vi "VI Tree.vi"   [LabVIEW 2020, in "NH Research Regenerative Test Series.lvlib"]
doc: "This instrument driver supports the NH Research 9400 Series AC/DC Power Module\".\n<B>Model Number</B> : 9400-4, 9400-8, 9400-12, 9400-24, 9400-36, 9400-48, 9400-64, 9400-96.\n\nThe VI Tree displays all the user-callable VIs of the instrument driver in an organized table."
uses:
  Drivers-Essentials/NH Research Regenerative Test Series.lvlib
  <instrlib>/NH Research Regenerative Test Series/Public/Data/Low Level/Fetch Array (Current).vi
  <instrlib>/NH Research Regenerative Test Series/Public/Data/Low Level/Fetch Waveform (Voltage).vi
  <instrlib>/NH Research Regenerative Test Series/Public/Data/Read Waveform (Voltage).vi
  <instrlib>/NH Research Regenerative Test Series/Public/Data/Read Array (Current).vi
  Data/Low Level/Fetch (Ave Current).vi
  Configure/Configure Slew Rate (Voltage).vi
  Action-Status/Query Slew Rate (Voltage).vi
  Action-Status/Reset Measurements (All).vi
  Data/Fetch Background Measurements (Basic).vi
  Drivers-Essentials/Read (Ave Current).vi
  Utility/Query Capabilities (Voltage).vi
panel:
  # "SEE DIAGRAM\nFOR VI TREE."
  # "NH Research, Inc. \n16601 Hale Avenue\nIrvine, CA 92606\n\nPhone:    (949) 474-3900\nEmail:      sales@nhresearch.com"
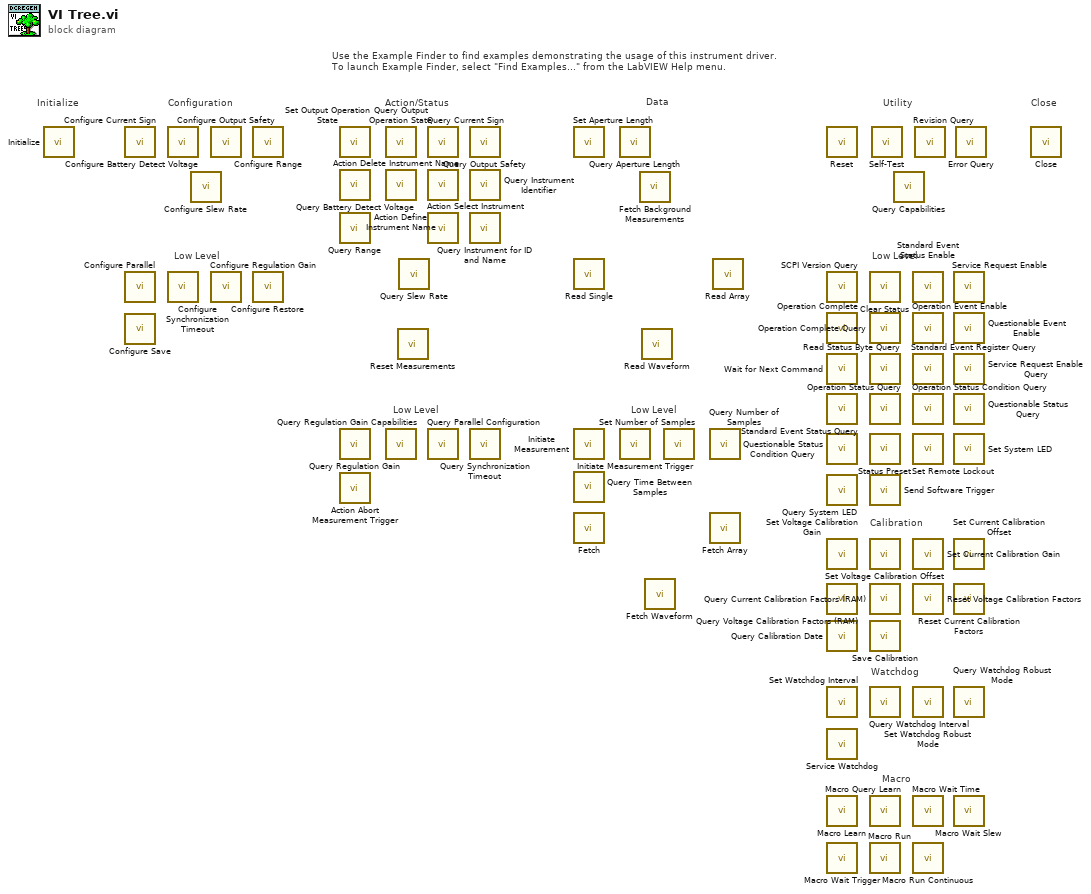
[diagram p0: block diagram]
diagram:
  # "Macro"
  # "Watchdog"
  # "Low Level"
  # "Calibration"
  # "Low Level"
  # "Low Level"
  # "Use the Example Finder to find examples demonstrating the usage of this instrument driver.\nTo launch Example Finder, select \"Find Examples...\" from the LabVIEW Help menu."
  # "Low Level"
  # "Configuration"
  # "Utility"
  # "Data"
  # "Action/Status"
  # "Close"
  # "Initialize"
  n1 = call <instrlib>:"Initialize.vi"() -> ()  [unwired: 14 in, 2 out]
  n2 = call <instrlib>:"Configure Current Sign.vi"() -> ()  [unwired: 14 in, 2 out]
  n3 = call <instrlib>:"Configure Parallel.vi"() -> ()  [unwired: 14 in, 2 out]
  n4 = call <instrlib>:"Configure Save.vi"() -> ()  [unwired: 14 in, 2 out]
  n5 = call "Configure Battery Detect Voltage.vi"() -> ()  [unwired: 14 in, 2 out]
  n6 = call <instrlib>:"Configure Synchronization Timeout.vi"() -> ()  [unwired: 14 in, 2 out]
  n7 = call-poly <instrlib>:"Configure Slew Rate.vi"() -> ()  [unwired: 14 in, 2 out]
  n8 = call <instrlib>:"Configure Output Safety.vi"() -> ()  [unwired: 14 in, 2 out]
  n9 = call <instrlib>:"Configure Regulation Gain.vi"() -> ()  [unwired: 14 in, 2 out]
  n10 = call "Configure Range.vi"() -> ()  [unwired: 14 in, 2 out]
  n11 = call <instrlib>:"Configure Restore.vi"() -> ()  [unwired: 14 in, 2 out]
  n12 = call <instrlib>:"Set Output Operation State.vi"() -> ()  [unwired: 14 in, 2 out]
  n13 = call <instrlib>:"Query Battery Detect Voltage.vi"() -> ()  [unwired: 13 in, 3 out]
  n14 = call "Query Range.vi"() -> ()  [unwired: 13 in, 3 out]
  n15 = call <instrlib>:"Query Regulation Gain.vi"() -> ()  [unwired: 13 in, 3 out]
  n16 = call <instrlib>:"Action Abort Measurement Trigger.vi"() -> ()  [unwired: 14 in, 2 out]
  n17 = call <instrlib>:"Query Output Operation State.vi"() -> ()  [unwired: 8 in, 8 out]
  n18 = call <instrlib>:"Action Define Instrument Name.vi"() -> ()  [unwired: 14 in, 2 out]
  n19 = call <instrlib>:"Query Regulation Gain Capabilities.vi"() -> ()  [unwired: 11 in, 5 out]
  n20 = call-poly <instrlib>:"Reset Measurements.vi"() -> ()  [unwired: 14 in, 2 out]
  n21 = call-poly <instrlib>:"Query Slew Rate.vi"() -> ()  [unwired: 13 in, 3 out]
  n22 = call "Query Current Sign.vi"() -> ()  [unwired: 13 in, 3 out]
  n23 = call <instrlib>:"Action Delete Instrument Name.vi"() -> ()  [unwired: 14 in, 2 out]
  n24 = call <instrlib>:"Action Select Instrument.vi"() -> ()  [unwired: 14 in, 2 out]
  n25 = call "Query Parallel Configuration.vi"() -> ()  [unwired: 13 in, 3 out]
  n26 = call "Query Output Safety.vi"() -> ()  [unwired: 13 in, 3 out]
  n27 = call <instrlib>:"Query Instrument Identifier.vi"() -> ()  [unwired: 13 in, 3 out]
  n28 = call <instrlib>:"Query Instrument for ID and Name.vi"() -> ()  [unwired: 12 in, 4 out]
  n29 = call "Query Synchronization Timeout.vi"() -> ()  [unwired: 13 in, 3 out]
  n30 = call <instrlib>:"Set Aperture Length.vi"() -> ()  [unwired: 14 in, 2 out]
  n31 = call-poly <instrlib>:"Read Single.vi"() -> ()  [unwired: 13 in, 3 out]
  n32 = call <instrlib>:"Initiate Measurement.vi"() -> ()  [unwired: 14 in, 2 out]
  n33 = call <instrlib>:"Query Time Between Samples.vi"() -> ()  [unwired: 13 in, 3 out]
  n34 = call-poly <instrlib>:"Fetch.vi"() -> ()  [unwired: 13 in, 3 out]
  n35 = call <instrlib>:"Query Aperture Length.vi"() -> ()  [unwired: 13 in, 3 out]
  n36 = call "Initiate Measurement Trigger.vi"() -> ()  [unwired: 14 in, 2 out]
  n37 = call-poly "Fetch Background Measurements.vi"() -> ()  [unwired: 13 in, 3 out]
  n38 = call-poly <instrlib>:"Read Waveform.vi"() -> ()  [unwired: 13 in, 3 out]
  n39 = call-poly <instrlib>:"Fetch Waveform.vi"() -> ()  [unwired: 13 in, 3 out]
  n40 = call <instrlib>:"Set Number of Samples.vi"() -> ()  [unwired: 14 in, 2 out]
  n41 = call <instrlib>:"Query Number of Samples.vi"() -> ()  [unwired: 13 in, 3 out]
  n42 = call-poly <instrlib>:"Fetch Array.vi"() -> ()  [unwired: 13 in, 3 out]
  n43 = call-poly <instrlib>:"Read Array.vi"() -> ()  [unwired: 13 in, 3 out]
  n44 = call <instrlib>:"Reset.vi"() -> ()  [unwired: 14 in, 2 out]
  n45 = call <instrlib>:"SCPI Version Query.vi"() -> ()  [unwired: 13 in, 3 out]
  n46 = call <instrlib>:"Operation Complete.vi"() -> ()  [unwired: 14 in, 2 out]
  n47 = call <instrlib>:"Wait for Next Command.vi"() -> ()  [unwired: 14 in, 2 out]
  n48 = call <instrlib>:"Standard Event Status Query.vi"() -> ()  [unwired: 13 in, 3 out]
  n49 = call <instrlib>:"Questionable Status Condition Query.vi"() -> ()  [unwired: 13 in, 3 out]
  n50 = call <instrlib>:"Query System LED.vi"() -> ()  [unwired: 13 in, 3 out]
  n51 = call "Set Voltage Calibration Gain.vi"() -> ()  [unwired: 14 in, 2 out]
  n52 = call <instrlib>:"Query Voltage Calibration Factors (RAM).vi"() -> ()  [unwired: 13 in, 3 out]
  n53 = call <instrlib>:"Query Calibration Date.vi"() -> ()  [unwired: 13 in, 3 out]
  n54 = call <instrlib>:"Set Watchdog Interval.vi"() -> ()  [unwired: 14 in, 2 out]
  n55 = call <instrlib>:"Service Watchdog.vi"() -> ()  [unwired: 14 in, 2 out]
  n56 = call "Macro Learn.vi"() -> ()  [unwired: 14 in, 2 out]
  n57 = call "Macro Wait Trigger.vi"() -> ()  [unwired: 14 in, 2 out]
  n58 = call <instrlib>:"Clear Status.vi"() -> ()  [unwired: 14 in, 2 out]
  n59 = call <instrlib>:"Operation Complete Query.vi"() -> ()  [unwired: 13 in, 3 out]
  n60 = call <instrlib>:"Read Status Byte Query.vi"() -> ()  [unwired: 13 in, 3 out]
  n61 = call <instrlib>:"Operation Status Query.vi"() -> ()  [unwired: 13 in, 3 out]
  n62 = call <instrlib>:"Status Preset.vi"() -> ()  [unwired: 14 in, 2 out]
  n63 = call "Send Software Trigger.vi"() -> ()  [unwired: 14 in, 2 out]
  n64 = call "Set Voltage Calibration Offset.vi"() -> ()  [unwired: 14 in, 2 out]
  n65 = call <instrlib>:"Query Current Calibration Factors (RAM).vi"() -> ()  [unwired: 13 in, 3 out]
  n66 = call <instrlib>:"Save Calibration.vi"() -> ()  [unwired: 14 in, 2 out]
  n67 = call <instrlib>:"Query Watchdog Interval.vi"() -> ()  [unwired: 13 in, 3 out]
  n68 = call "Macro Query Learn.vi"() -> ()  [unwired: 13 in, 3 out]
  n69 = call "Macro Run.vi"() -> ()  [unwired: 14 in, 2 out]
  n70 = call <instrlib>:"Self-Test.vi"() -> ()  [unwired: 13 in, 3 out]
  n71 = call-poly <instrlib>:"Query Capabilities.vi"() -> ()  [unwired: 13 in, 3 out]
  n72 = call <instrlib>:"Standard Event Status Enable.vi"() -> ()  [unwired: 14 in, 2 out]
  n73 = call <instrlib>:"Operation Event Enable.vi"() -> ()  [unwired: 14 in, 2 out]
  n74 = call <instrlib>:"Standard Event Register Query.vi"() -> ()  [unwired: 13 in, 3 out]
  n75 = call <instrlib>:"Operation Status Condition Query.vi"() -> ()  [unwired: 13 in, 3 out]
  n76 = call <instrlib>:"Set Remote Lockout.vi"() -> ()  [unwired: 14 in, 2 out]
  n77 = call <instrlib>:"Set Current Calibration Gain.vi"() -> ()  [unwired: 14 in, 2 out]
  n78 = call <instrlib>:"Reset Voltage Calibration Factors.vi"() -> ()  [unwired: 14 in, 2 out]
  n79 = call <instrlib>:"Set Watchdog Robust Mode.vi"() -> ()  [unwired: 14 in, 2 out]
  n80 = call "Macro Wait Time.vi"() -> ()  [unwired: 14 in, 2 out]
  n81 = call "Macro Run Continuous.vi"() -> ()  [unwired: 14 in, 2 out]
  n82 = call <instrlib>:"Revision Query.vi"() -> ()  [unwired: 11 in, 5 out]
  n83 = call <instrlib>:"Service Request Enable.vi"() -> ()  [unwired: 14 in, 2 out]
  n84 = call <instrlib>:"Questionable Event Enable.vi"() -> ()  [unwired: 14 in, 2 out]
  n85 = call <instrlib>:"Service Request Enable Query.vi"() -> ()  [unwired: 13 in, 3 out]
  n86 = call <instrlib>:"Questionable Status Query.vi"() -> ()  [unwired: 13 in, 3 out]
  n87 = call <instrlib>:"Set System LED.vi"() -> ()  [unwired: 14 in, 2 out]
  n88 = call "Set Current Calibration Offset.vi"() -> ()  [unwired: 14 in, 2 out]
  n89 = call <instrlib>:"Reset Current Calibration Factors.vi"() -> ()  [unwired: 14 in, 2 out]
  n90 = call <instrlib>:"Query Watchdog Robust Mode.vi"() -> ()  [unwired: 13 in, 3 out]
  n91 = call "Macro Wait Slew.vi"() -> ()  [unwired: 14 in, 2 out]
  n92 = call "Error Query.vi"() -> ()  [unwired: 12 in, 4 out]
  n93 = call <instrlib>:"Close.vi"() -> ()  [unwired: 15 in, 1 out]
